vi "Agilent 532XX Series Limit Test.vi"() -> ()   [LabVIEW 2021]
doc: "This example shows how to acquire limit test result using the VIs of the driver."
uses:
  <instrlib>/Agilent 532XX Series/Public/Configure/Measurement/Configure Measurement (Frequency).vi
  <instrlib>/Agilent 532XX Series/Agilent 532XX Series.lvlib
panel:
  in  "Frequency Estimate (10E+6 Hz)":dbl=10000000.0 format="%^#_6g"
  in  "Channel (1:Channel 1)":i32(ring)=1 items=["Channel 1"=1, "Channel 2"=2, "Channel 3"=3]
  in  "Frequency Resolution (1 Hz)":dbl=1.0
  in  "Lower Limit Value (0 Hz)":dbl
  in  "Upper Limit Value (0 Hz)":dbl
  out "Upper Limit Test Fail ?":bool
  out "Lower Limit Test Fail ?":bool
  in  "Number of Measurement (100)":u32=100
  in  "Timeout (10000 ms)":u32=10000
  in  "VISA resource name":refnum<visa-resource-name>
  # "(c) 2010-2015 National Instruments.  ALL RIGHTS RESERVED."
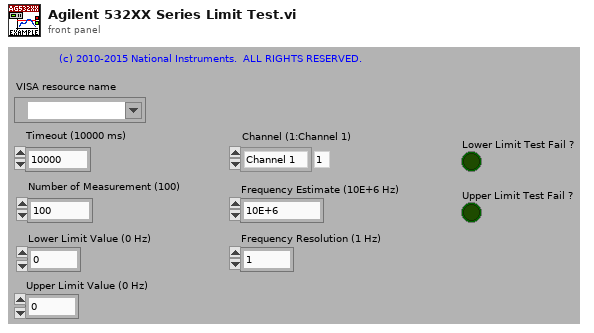
[diagram p1: front panel]
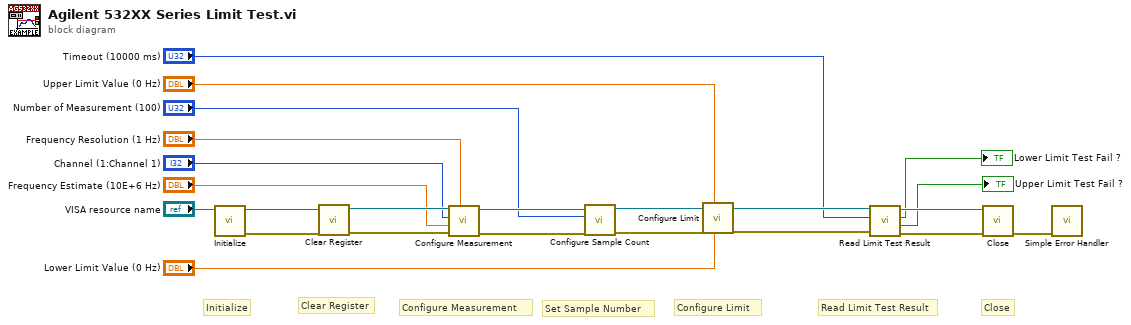
[diagram p0: block diagram]
diagram:
  # "Clear Register"
  # "Configure Limit"
  # "Set Sample Number"
  # "Close"
  # "Read Limit Test Result"
  # "Initialize"
  # "Configure Measurement"
  n1 = call <instrlib>:"Initialize.vi"("VISA resource name"="VISA resource name") -> ("error out"=w15:errorcluster, "VISA resource name out"=w16:refnum<visa-resource-name>)  [unwired: 3 in, 6 out]
  n2 = call <instrlib>:"Clear Register .vi"("error in (no error)"=w15, "VISA resource name"=w16) -> ("error out"=w17:errorcluster, "VISA resource name out"=w18:refnum<visa-resource-name>)  [unwired: 8 out]
  n3 = call-poly <instrlib>:"Configure Measurement.vi"("Frequency Resolution (1 Hz)"="Frequency Resolution (1 Hz)", "error in (no error)"=w17, "Frequency Estimate (10E+6 Hz)"="Frequency Estimate (10E+6 Hz)", "Channel (1:Channel 1)"="Channel (1:Channel 1)", "VISA resource name"=w18) -> ("error out"=w20:errorcluster, "VISA resource name out"=w21:refnum<visa-resource-name>)  [unwired: 5 out]
  n4 = call <instrlib>:"Configure Sample Count.vi"("error in (no error)"=w20, "Sample Count (1)"="Number of Measurement (100)", "VISA resource name"=w21) -> ("error out"=w13:errorcluster, "VISA resource name out"=w14:refnum<visa-resource-name>)  [unwired: 7 out]
  n5 = call <instrlib>:"Configure Limit.vi"("Lower Limit Value (0 Hz)"="Lower Limit Value (0 Hz)", "Upper Limit Value (0 Hz)"="Upper Limit Value (0 Hz)", "error in (no error)"=w13, "VISA resource name"=w14) -> ("error out"=w9:errorcluster, "VISA resource name out"=w10:refnum<visa-resource-name>)  [unwired: 2 in, 4 out]
  n6 = call <instrlib>:"Read Limit Test Result.vi"("error in (no error)"=w9, "Timeout (10000 ms)"="Timeout (10000 ms)", "VISA resource name"=w10) -> ("error out"=w6:errorcluster, "Upper Limit Test Fail?"=→"Upper Limit Test Fail ?":bool, "Lower Limit Test Fail?"=→"Lower Limit Test Fail ?":bool, "VISA resource name out"=w7:refnum<visa-resource-name>)  [unwired: 5 out]
  n7 = call <instrlib>:"Close.vi"("error in (no error)"=w6, "VISA resource name"=w7) -> ("error out"=w22:errorcluster)  [unwired: 9 out]
  n8 = call <vilib>:"Simple Error Handler.vi"("error in (no error)"=w22) -> ()  [unwired: 1 in, 8 out]
